vi "KB-RS232-OpenVISA.vi"(9 "比特":string, 10 "波特率":string, 11 "VISA资源名称":refnum<visa-resource-name>="COM1") -> (3 "VISA resource name out":refnum<visa-resource-name> caption="VISA资源名称输出")   [LabVIEW 2017]
uses:
  <vilib>/Instr/_visa.llb/VISA Configure Serial Port (Instr).vi
  Program Files (x86)/National Instruments/LabVIEW 2015/examples/Instrument IO/Serial/support/Serial - Settings.ctl
panel:
  out "error out":errorcluster caption="错误输出"
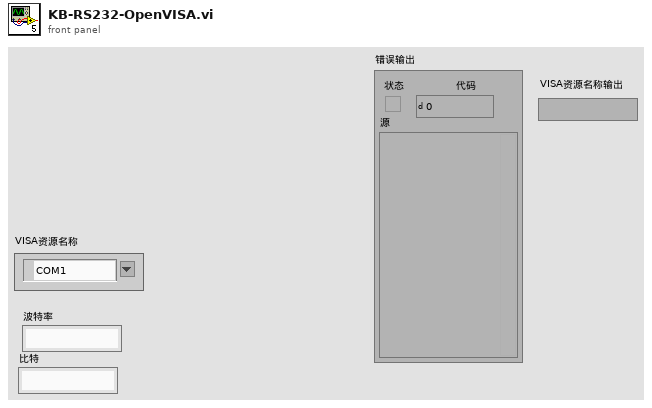
[diagram p1: front panel]
types:
  T1 = typedef "Serial - Settings.ctl" = cluster{"波特率":u32, "数据比特":u16, "奇偶":enum16{"None", "Odd", "Even", "Mark", "Space"}, "停止位":u16, "流控制":u16}
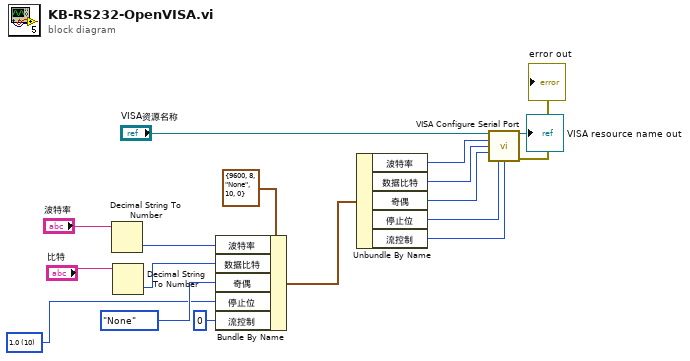
[diagram p0: block diagram]
diagram:
  w1 = u16 10 items=["1.0"=10, "1.5"=15, "2.0"=20] ("停止位")
  n1 = Decimal String To Number(string="波特率") -> (number=w9:i32)  [unwired: 2 in, 1 out]
  n2 = Decimal String To Number(string="比特") -> (number=w7:i32)  [unwired: 2 in, 1 out]
  n3 = Bundle By Name(cluster=T1 {"波特率"=9600, "数据比特"=8, "奇偶"=enum."None", "停止位"=10, "流控制"=0} ("串口设置"), "波特率"=w9, "数据比特"=w7, "奇偶"=enum16{"None", "Odd", "Even", "Mark", "Space"}."None", "停止位"=w1, "流控制"=u16 0) -> (w3:T1)
  n4 = Unbundle By Name(w3) -> ("波特率"=w16:u32, "数据比特"=w15:u16, "奇偶"=w14:enum16{"None", "Odd", "Even", "Mark", "Space"}, "停止位"=w13:u16, "流控制"=w12:u16)
  n5 = call-poly "VISA Configure Serial Port"("VISA resource name"="VISA资源名称", "baud rate (9600)"=w16, "data bits (8)"=w15, "parity (0:none)"=w14, "stop bits (10: 1 bit)"=w13, "flow control (0:none)"=w12) -> ("VISA resource name out"=→"VISA resource name out":refnum<visa-resource-name>, "error out"=→"error out":errorcluster)  [unwired: 3 in, 5 out]
